vi "VI Analyzer Status.vi"(0 "VI Analyzer Task in":T1) -> ()   [LabVIEW 2015, in "Model.lvlib" / "Model.lvclass"]
uses:
  <resource>/Framework/Providers/TomsToolsDocumentationTool/Source Code/Model/Model.lvclass
  <vilib>/addons/analyzer/_analyzerctrls.llb/VIAnAPI Ref.ctl
  <vilib>/addons/analyzer/NI_VIAnalyzerTKVIs.lvlib
panel:
  out "Test Progress":u8(slide) scale=0.0..100.0
  in  "Abort Analysis":bool
  # "Developer note:\nAbort Analysis is not available in LV15"
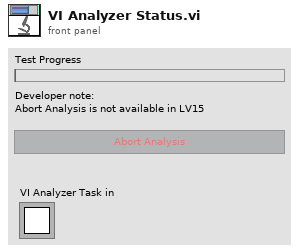
[diagram p1: front panel]
types:
  T1 = typedef "VIAnAPI Ref.ctl" = refnum<k1>
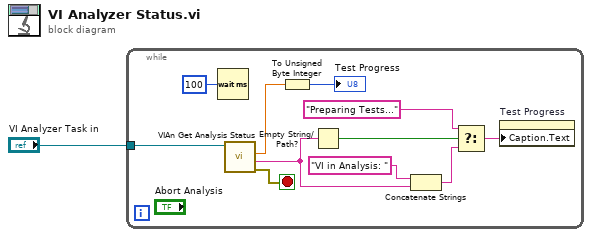
[diagram p0: block diagram]
diagram:
  n1 = while {
    tunnel: "VI Analyzer Task in" -> [w8]
    stop <- w11 stop-if-true
    n2 = Wait (ms)(milliseconds to wait=u32 100) -> ()  [unwired: 1 out]
    n3 = call <vilib>:"VIAn Get Analysis Status.vi"("VI Analyzer Task in"=w8) -> ("error out"=w11:errorcluster, "VI in Analysis"=w4:string, "Percent Complete"=w10:dbl)  [unwired: 2 in, 6 out]
    n4 = To Unsigned Byte Integer(number=w10) -> (unsigned 8bit integer=→"Test Progress":u8)
    n5 = Empty String/Path?(string/path=w4) -> (empty?=w7:bool)
    n6 = Concatenate Strings("VI in Analysis: ", w4) -> (w2:string)
    n7 = Select(t="Preparing Tests...", s=w7, f=w2) -> (s? t:f=w6:string)
    n8 = property on="Test Progress" class="Slide (strict)"("Caption.Text"=w6) -> ()  [unwired: 2 in, 2 out]
  }
